vi "String Indicator BG Color.vi"(10 "BG Color":u32(colorbox), 11 "Dev Panel in":refnum<class "Dev Panel.lvclass">) -> (0 "error out":errorcluster)   [LabVIEW 2021, in "Dev Panel.lvclass"]
uses:
  Dev Panel.lvclass
  Dev Panel.lvclass/Dev Panel.ctl
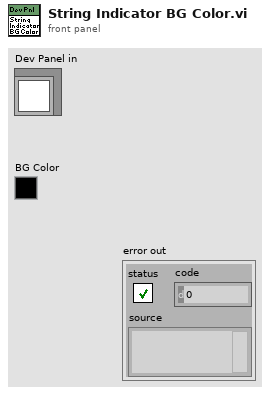
[diagram p1: front panel]
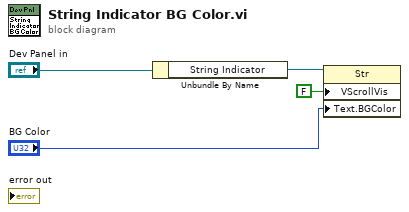
[diagram p0: block diagram]
diagram:
  n1 = Unbundle By Name("Dev Panel in") -> ("String Indicator"=w3:refnum<vi>)
  n2 = property class="Str"(reference=w3, "VScrollVis"=FALSE ("Vertical Scrollbar Visible"), "Text.BGColor"="BG Color") -> ()  [unwired: 1 in, 2 out]
